vi "Read GPIO Bank.vi"(0 "fpga interface in":refnum<k20>, 5 "gpio bank select":T1, 11 "error in (no error)":errorcluster) -> (4 "fpga interface out":refnum<k20>, 6 "gpio bank output":T2, 15 "error out":errorcluster)   [LabVIEW 2023, in "GettingStarted_Common_148X_Host.lvlib"]
uses:
  GettingStarted_Common_148X_Host.lvlib
  <instrlib>/FlexRIO/CSI-2/v2/FPGA/Types/GPIO Bank.ctl
  FPGA/Common/Types/SerDes Identifier.ctl
  Types/148x_Common_FPGA_Reference.ctl
  <vilib>/rvi/errors/niLvFpgaAdjustHostInterfaceError.vi
  <vilib>/rvi/interface/nirviReadWriteControl/nirviReadWriteControl.xnode
  NiFpgaLv.dll
  <vilib>/rvi/interface/Simulation/niFpgaSimulationCallBeginRW.vi
  FPGA/Common/GettingStarted_Common_148X_FPGA.lvlib
  <instrlib>/FlexRIO/CSI-2/v2/FPGA/NI CSI-2 API FPGA v2.lvlib
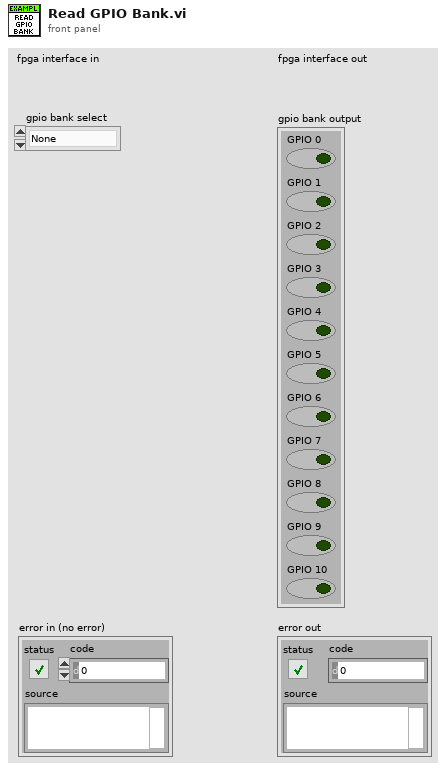
[diagram p1: front panel]
types:
  T1 = typedef "GettingStarted_Common_148X_FPGA.lvlib/SerDes Identifier.ctl" = enum8{"None", "SI 0 Deserializer", "SI 1 Deserializer", "SI 2 Deserializer", "SI 3 Deserializer", "SI 4 Deserializer", "SI 5 Deserializer", "SI 6 Deserializer", "SI 7 Deserializer", "SO 0 Serializer", "SO 1 Serializer", "SO 2 Serializer", "SO 3 Serializer", "SO 4 Serializer", "SO 5 Serializer", "SO 6 Serializer", "SO 7 Serializer", "SI 0 SI 1 Deserializer", "SI 2 SI 3 Deserializer", "SI 4 SI 5 Deserializer", "SI 6 SI 7 Deserializer"}
  T2 = typedef "NI CSI-2 API FPGA v2.lvlib/GPIO Bank.ctl" = cluster{"GPIO 0":bool, "GPIO 1":bool, "GPIO 2":bool, "GPIO 3":bool, "GPIO 4":bool, "GPIO 5":bool, "GPIO 6":bool, "GPIO 7":bool, "GPIO 8":bool, "GPIO 9":bool, "GPIO 10":bool}
  T3 = typedef "GettingStarted_Common_148X_Host.lvlib/148x_Common_FPGA_Reference.ctl" = refnum<k20>
  T4 = cluster{"GPIO 0":bool, "GPIO 1":bool, "GPIO 2":bool, "GPIO 3":bool, "GPIO 4":bool, "GPIO 5":bool, "GPIO 6":bool, "GPIO 7":bool, "GPIO 8":bool, "GPIO 9":bool, "GPIO 10":bool}
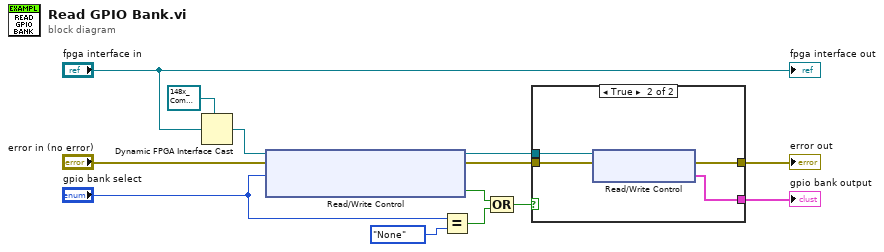
[diagram p0: block diagram]
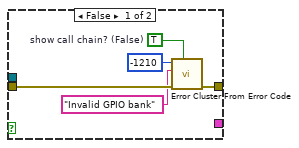
[diagram p2: hidden frame]
diagram:
  n1 = Dynamic FPGA Interface Cast(Session In=T3 refnum ("FPGA VI Reference Out"), Type="fpga interface in") -> (Session Out=w12:T3)
  n2 = xnode "Read/Write Control"("FPGA VI Reference In"=w12, "error in"="error in (no error)", "gpio bank input select"="gpio bank select") -> ("FPGA VI Reference Out"=w7:T3, "error out"=w9:errorcluster, "serdes gpio bank input select valid"=w2:bool)
  n3 = Equal?(x="gpio bank select", y=SerDes_Identifier."None") -> (x = y?=w3:bool)
  n4 = Compound Arithmetic op=OR(w2, w3) -> (w1:bool)
  n5 = case shown="True" w1 {
    tunnel: w9 -> [w18 w22]
    tunnel: [w17 w20] -> w8
    tunnel: w7 -> [_ w21]
    tunnel: [_ w19] -> w6
    frame False {
      w14 = TRUE  # show call chain? (False)
      n6 = call <vilib>:"Error Cluster From Error Code.vi"("show call chain? (False)"=w14, "error in (no error)"=w18, "error message (\"\")"="Invalid GPIO bank" ("error message (\"\")"), "error code (0)"=-1210) -> ("error out"=w17:errorcluster)  [unwired: 5 in]
    }
    frame True {
      n7 = xnode "Read/Write Control"("FPGA VI Reference In"=w21, "error in"=w22) -> ("error out"=w20:errorcluster, "gpio bank input"=w19:T4)  [unwired: 1 out]
    }
  }
  "error out" <- w8
  "gpio bank output" <- w6
  "fpga interface out" <- "fpga interface in"
